vi "Shutdown.vi"(8 "error in (no error)":errorcluster, 11 "Temp Chamber in":refnum<class "Temp Chamber.lvclass">) -> (0 "error out":errorcluster, 3 "Temp Chamber out":refnum<class "Temp Chamber.lvclass">)   [LabVIEW 2018, in "Temp Chamber.lvlib" / "Temp Chamber.lvclass"]
uses:
  Temp Chamber.lvclass
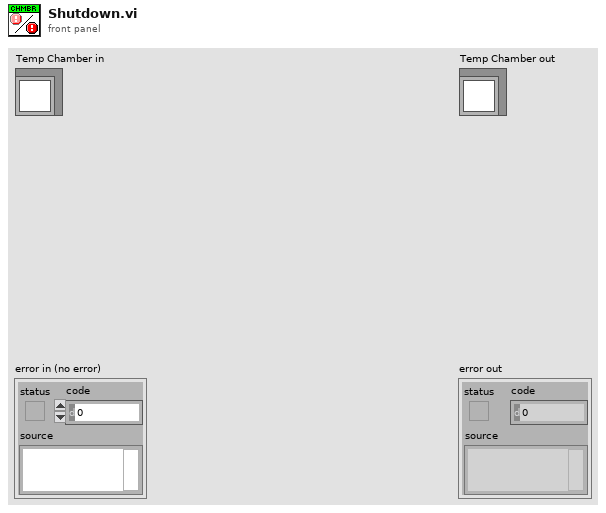
[diagram p1: front panel]
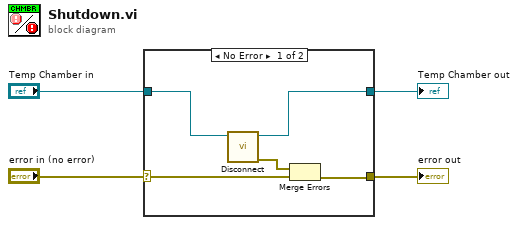
[diagram p0: block diagram]
diagram:
  n1 = case shown="No Error" "error in (no error)" {
    selector: "error in (no error)" -> [w8 w11]
    tunnel: [w7 w11] -> w3
    tunnel: [w5 w10] -> w1
    tunnel: "Temp Chamber in" -> [w6 w10]
    frame No Error {
      n2 = call-dynamic "Disconnect.vi"("Temp Chamber in"=w6) -> ("error out"=w9:errorcluster, "Temp Chamber out"=w5:refnum<class "Temp Chamber.lvclass">)  [unwired: 9 in]
      n3 = Merge Errors(w9, w8) -> (w7:errorcluster)
    }
    frame Error {
    }
  }
  "error out" <- w3
  "Temp Chamber out" <- w1
